vi "Read Attributes.vi"(11 "Generate Report Msg":refnum<class "Generate Report Msg.lvclass">) -> (2 "Payload":cluster{"Generate Report":bool})   [LabVIEW 2017, in "User Interface.lvlib" / "Generate Report Msg.lvclass"]
uses:
  Generate Report Msg.lvclass
  Generate Report Msg.lvclass/Generate Report Msg.ctl
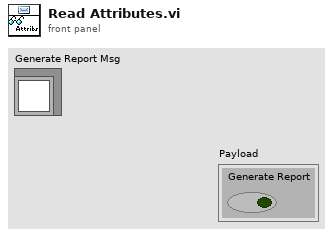
[diagram p1: front panel]
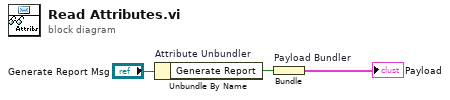
[diagram p0: block diagram]
diagram:
  n1 = Unbundle By Name "Attribute Unbundler"("Generate Report Msg") -> ("Generate Report"=w1:bool)
  n2 = Bundle "Payload Bundler"("Generate Report"=w1) -> (→"Payload":cluster{"Generate Report":bool})  [unwired: 1 in]
